vi "DS BaseActor StartStop Polling.vi"() -> ()   [LabVIEW 2016, in "CS++Utilities.lvlib"]
doc: "Activate or deactivate CS++PVProxy when using DataSocket."
uses:
  CS++Utilities.lvlib
panel:
  in  "Start? (T)":bool
  in  "Polling StartStop URL":string="dstp://localhost/CSPP_Core_SV/myBaseActor_PollingStartStop"
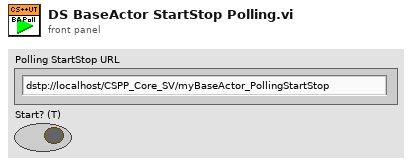
[diagram p1: front panel]
types:
  T1 = enum16{"Read", "Write", "ReadWrite", "BufferedRead", "BufferedReadWrite"}
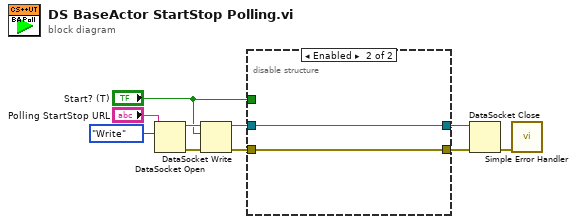
[diagram p0: block diagram]
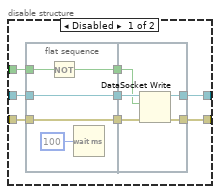
[diagram p2: hidden frame]
diagram:
  n1 = DataSocket Open(10:T1."Write" ("mode"), 11:"Polling StartStop URL") -> (0:w9:errorcluster, 3:w7:refnum<k13>)  [unwired: 2 in]
  n2 = DataSocket Write(8:w9, 10:"Start? (T)", 11:w7) -> (0:w4:errorcluster, 3:w3:refnum<k13>)  [unwired: 1 in, 1 out]
  n3 = disable-structure shown="Enabled" {
    disable-tunnel: [w15 w29] -> w5
    disable-tunnel: w4 -> [w14 w29]
    disable-tunnel: w3 -> [w13 w30]
    disable-tunnel: [w12 w30] -> w2
    disable-tunnel: "Start? (T)" -> [w11 _]
    frame Disabled {
      n4 = flat-sequence {
        tunnel: w13 -> [w22]
        tunnel: w14 -> [w23]
        tunnel: [w23] -> w18
        tunnel: [w22] -> w17
        tunnel: [w20] -> w16
        tunnel: w11 -> [w19]
        tunnel: [w28] -> w15
        tunnel: [w24] -> w12
        tunnel: w18 -> [w27]
        tunnel: w17 -> [w26]
        tunnel: w16 -> [w25]
        frame #0 {
          n5 = Not(x=w19) -> (.not. x?=w20:bool)
          n6 = Wait (ms)(milliseconds to wait=u32 100) -> ()  [unwired: 1 out]
        }
        frame #1 {
          n7 = DataSocket Write(8:w27, 10:w25, 11:w26) -> (0:w28:errorcluster, 3:w24:refnum<k13>)  [unwired: 1 in, 1 out]
        }
      }
    }
    frame Enabled {
    }
  }
  n8 = DataSocket Close(8:w5, 11:w2) -> (0:w6:errorcluster)  [unwired: 1 in, 1 out]
  n9 = call <vilib>:"Simple Error Handler.vi"("error in (no error)"=w6) -> ()  [unwired: 4 in, 5 out]
